vi "FRAS Filtre.vi"(0 "CdG(t)":dbl[](array[numeric]), 7 "Tableau 2":dbl[](array[numeric]), 11 "Gain_int":dbl) -> (8 "Tableau":dbl[](array[numeric]))   [LabVIEW 2020]
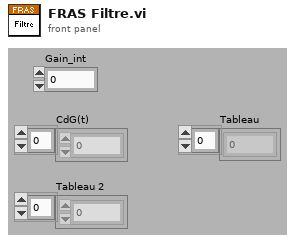
[diagram p1: front panel]
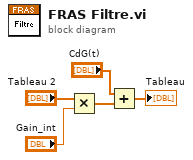
[diagram p0: block diagram]
diagram:
  n1 = Multiply(x="Tableau 2", y="Gain_int") -> (x*y=w4:dbl[])
  n2 = Add(x="CdG(t)", y=w4) -> (x+y=→"Tableau":dbl[])
